vi "RT Proccesing.vi"(8 "error in (no error)":errorcluster, 10 "info":cluster{"File path":T4, "Cfg ":T5} {"Cfg"."Offset_rueda WS 2" format="%.27g"; "Cfg"."Offset_rueda WS 1" format="%.27g"; "Cfg"."Frecuencia de muestreo y módulo CRIO" items=["51.200 kS/s (NI 9234)"=1, "25.600 kS/s (NI 9234)"=2, "17.067 kS/s (NI 9234)"=3, "12.800 kS/s (NI 9234)"=4, "10.240 kS/s (NI 9234)"=5, "8.533 kS/s (NI 9234)"=6, "7.314 kS/s (NI 9234)"=7, "6.400 kS/s (NI 9234)"=8, "5.689 kS/s (NI 9234)"=9, "5.120 kS/s (NI 9234)"=10, "4.654 kS/s (NI 9234)"=11, "4.267 kS/s (NI 9234)"=12, "3.938 kS/s (NI 9234)"=13, "3.657 kS/s (NI 9234)"=14, "3.413 kS/s (NI 9234)"=15, "3.200 kS/s (NI 9234)"=16, "3.012 kS/s (NI 9234)"=17, "2.845 kS/s (NI 9234)"=18, "2.695 kS/s (NI 9234)"=19, "2.560 kS/s (NI 9234)"=20, "2.438 kS/s (NI 9234)"=21, "2.328 kS/s (NI 9234)"=22, "2.226 kS/s (NI 9234)"=23, "2.133 kS/s (NI 9234)"=24, "2.048 kS/s (NI 9234)"=25, "1.969 kS/s (NI 9234)"=26, "1.896 kS/s (NI 9234)"=27, "1.829 kS/s (NI 9234)"=28, "1.765 kS/s (NI 9234)"=29, "1.707 kS/s (NI 9234)"=30, "1.652 kS/s (NI 9234)"=31]}, 11 "Message Queues in":T7) -> (0 "error out":errorcluster)   [LabVIEW 2015]
uses:
  support/Message Queue/All Message Queues.ctl
  support/Message Queue/Message Cluster.ctl
  controls/File paths.ctl
  controls/Cfg_parameters.ctl
  <vilib>/LabVIEW Targets/FPGA/cRIO/shared/nicrio_ModuleControls/nicrio_cRIO-9234_DataRatesRing2.ctl
  controls/Flota.ctl
  controls/Tags.ctl
  controls/Processing data.ctl
  support/Message Queue/Enqueue Message (Single).vi
  <vilib>/Utility/file.llb/Write Delimited Spreadsheet (string).vi
  <vilib>/Utility/error.llb/Error Cluster From Error Code.vi
  <vilib>/ErrorRing/Error Ring.xnode
  support/Message Queue/Message Queue.lvlib
  AURA_Wheel/Json2Labv.lvlib
  AURA_Wheel/AuraWheelAPI/AuraWheel.lvlib
panel:
  out "Response headers":string
  out "data":cluster{"status":string}
  in  "Procesado":T1
  in  "TAGs":T2
  in  "Flota":T3
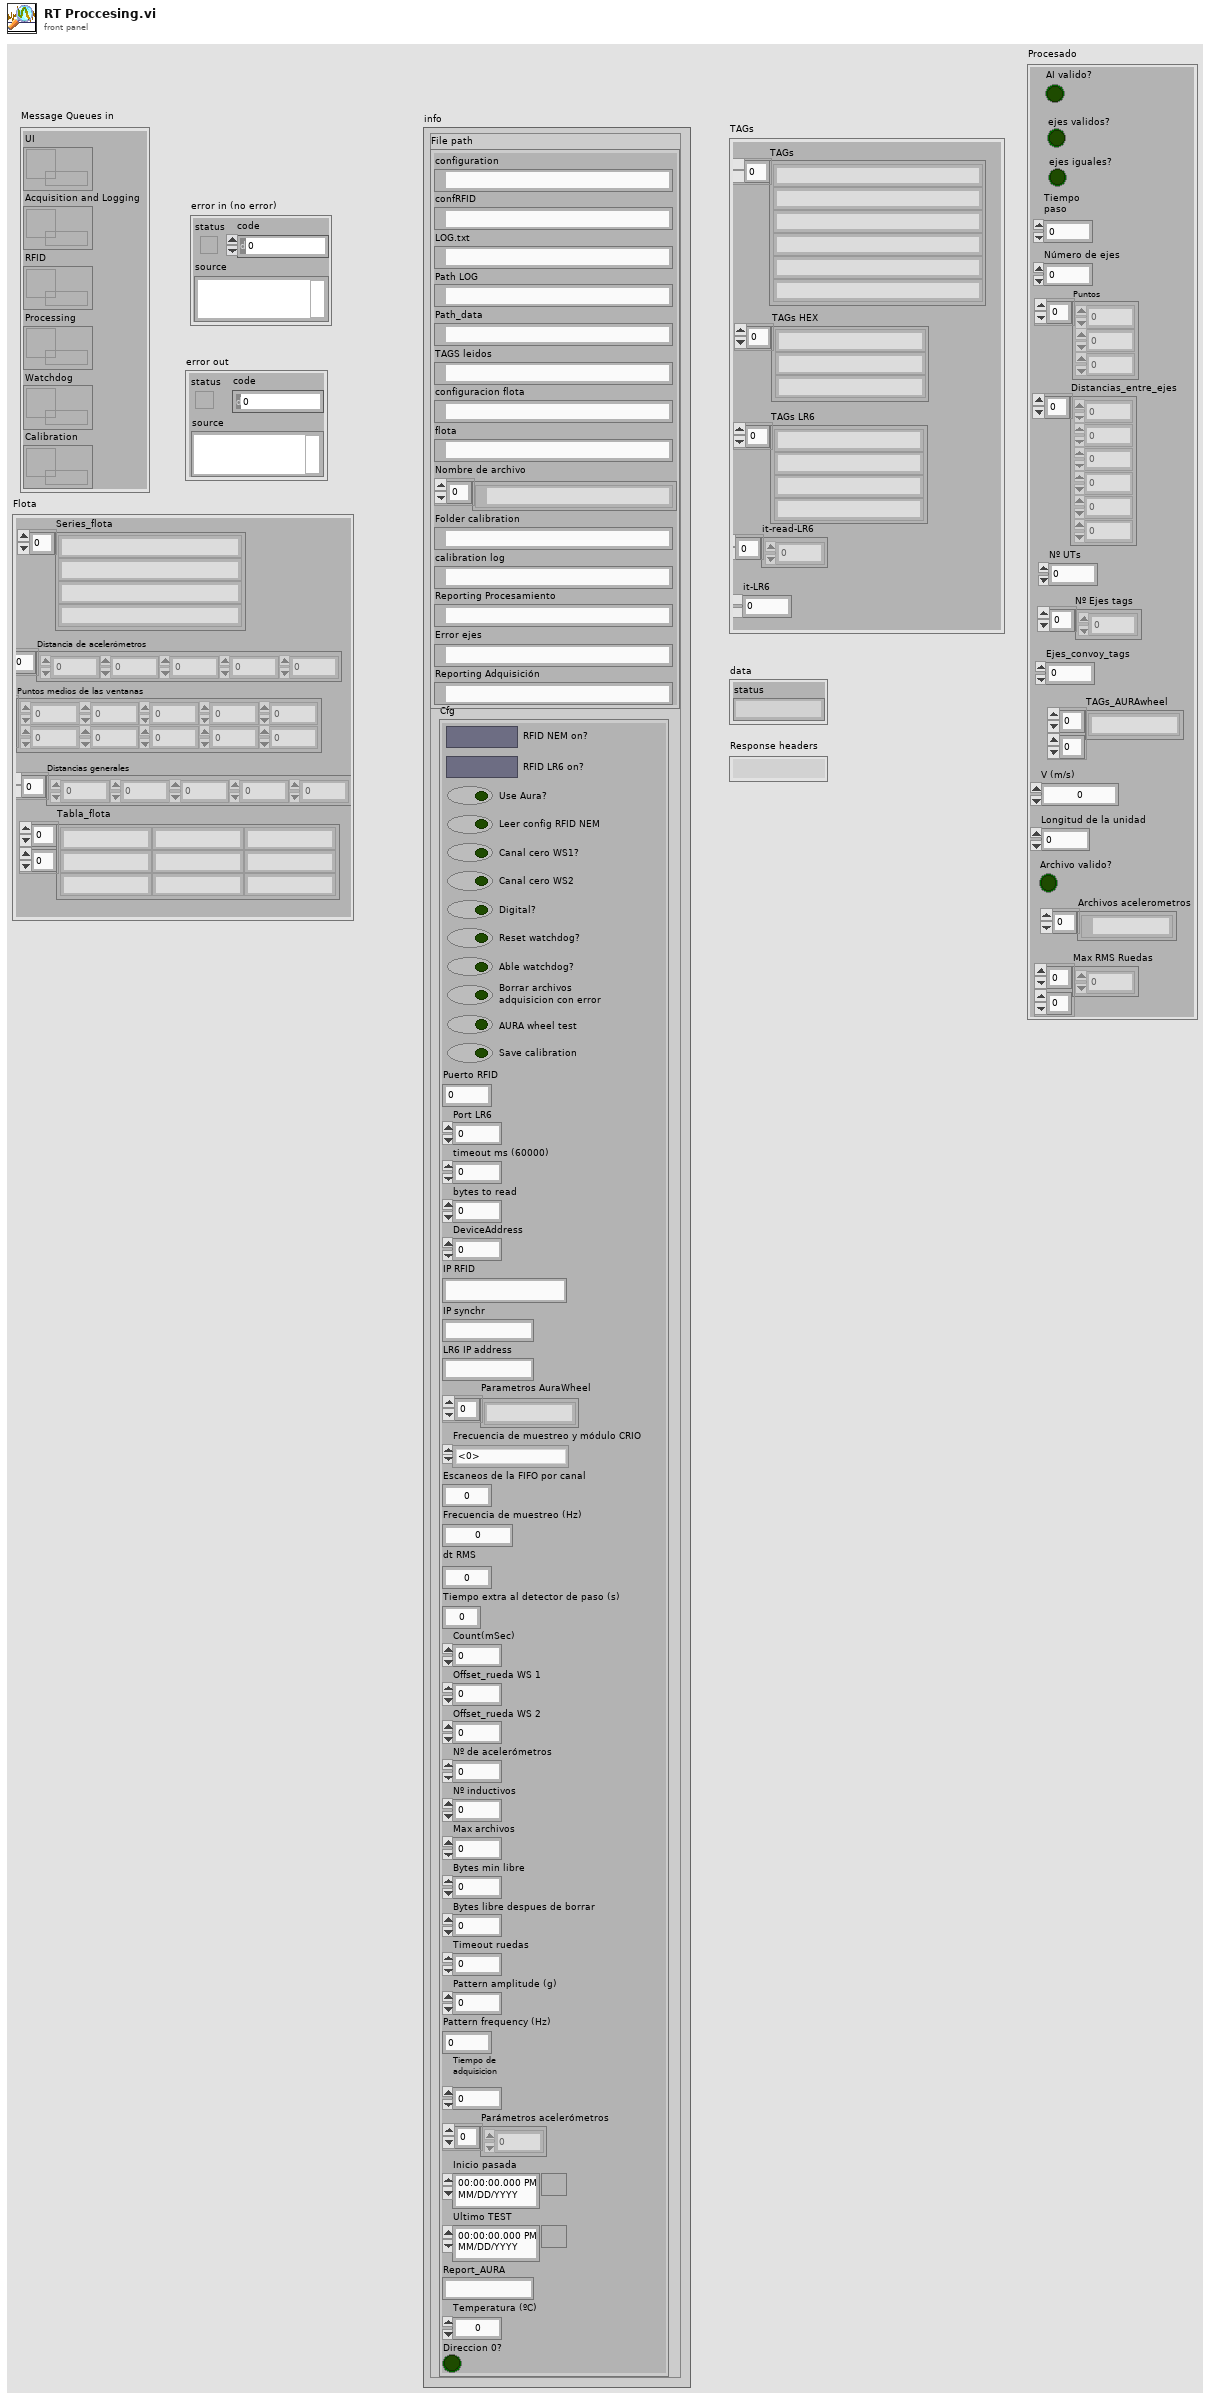
[diagram p1: front panel]
types:
  T1 = typedef "Processing data.ctl" = cluster{"AI valido?":bool, "Tiempo\npaso":dbl, "Puntos":sgl[], "Número de ejes":i32, "ejes validos?":bool, "ejes iguales?":bool, "Distancias_entre_ejes":dbl[], "Nº UTs":i32, "Nº Ejes tags":i32[], "Ejes_convoy_tags":i32, "TAGs_AURAwheel":string[][], "V (m/s)":dbl, "Longitud de la unidad":dbl, "Archivo valido?":bool, "Archivos acelerometros":path[], "Max RMS Ruedas":dbl[][]}
  T2 = typedef "Tags.ctl" = cluster{"TAGs":string[], "TAGs HEX":string[], "TAGs LR6":string[], "it-read-LR6":i32[], "it-LR6":i32}
  T3 = typedef "Flota.ctl" = cluster{"Series_flota":string[], "Distancia de acelerómetros":dbl[], "Puntos medios de las ventanas":dbl[][], "Distancias generales":dbl[], "Tabla_flota":string[][]}
  T4 = typedef "File paths.ctl" = cluster{"configuration":path, "confRFID":path, "LOG.txt":path, "Path LOG":path, "Path_data":path, "TAGS leidos":path, "configuracion flota":path, "flota":path, "Nombre de archivo":path[], "Folder calibration":path, "calibration log":path, "Reporting Procesamiento":path, "Error ejes":path, "Reporting Adquisición":path}
  T5 = typedef "Cfg_parameters.ctl" = cluster{"RFID NEM on?":bool, "RFID LR6 on?":bool, "Use Aura?":bool, "Leer config RFID NEM":bool, "Canal cero WS1?":bool, "Canal cero WS2 ":bool, "Digital?":bool, "Reset watchdog?":bool, "Able watchdog?":bool, "Borrar archivos\nadquisicion con error":bool, "AURA wheel test":bool, "Save calibration":bool, "Puerto RFID":u16, "Port LR6":u16, "timeout ms (60000)":i32, "bytes to read":i32, "DeviceAddress":u8, "IP RFID":string, "IP synchr":string, "LR6 IP address":string, "Parametros AuraWheel":string[], "Frecuencia de muestreo y módulo CRIO":T6, "Escaneos de la FIFO por canal":u32, "Frecuencia de muestreo (Hz)":dbl, "dt RMS":dbl, "Tiempo extra al detector de paso (s)":dbl, "Count(mSec)":u32, "Offset_rueda WS 1":fxp<+/-,24,-4>, "Offset_rueda WS 2":fxp<+/-,24,-4>, "Nº de acelerómetros":i32, "Nº inductivos":i32, "Max archivos":u32, "Bytes min libre":u32, "Bytes libre despues de borrar":u32, "Timeout ruedas":dbl, "Pattern amplitude (g)":dbl, "Pattern frequency (Hz)":dbl, "Tiempo de adquisicion\n":dbl, "Parámetros acelerómetros":dbl[], "Inicio pasada":timestamp, "Ultimo TEST":timestamp, "Report_AURA":string, "Temperatura (ºC)":dbl, "Direccion 0?":bool}
  T6 = typedef "nicrio_cRIO-9234_DataRatesRing2.ctl" = u8
  T7 = typedef "Message Queue.lvlib/All Message Queues.ctl" = cluster{"UI":refnum<queue>, "Acquisition and Logging":refnum<queue>, "RFID":refnum<queue>, "Processing":refnum<queue>, "Watchdog":refnum<queue>, "Calibration":refnum<queue>}
  T8 = enum16{"big-endian, network order", "native, host order", "little-endian"}
  T9 = cluster{"g_ts":dbl, "p_sp":dbl, "p_tp":dbl, "p_tg":cluster{"tg_n":dbl, "tg_t":string}[], "p_ax":cluster{"ax_n":dbl, "ax_sp":dbl, "ax_wh":cluster{"wh_p":dbl, "wh_a1":dbl, "wh_a2":dbl, "wh_a3":dbl, "wh_a4":dbl}[]}[]}
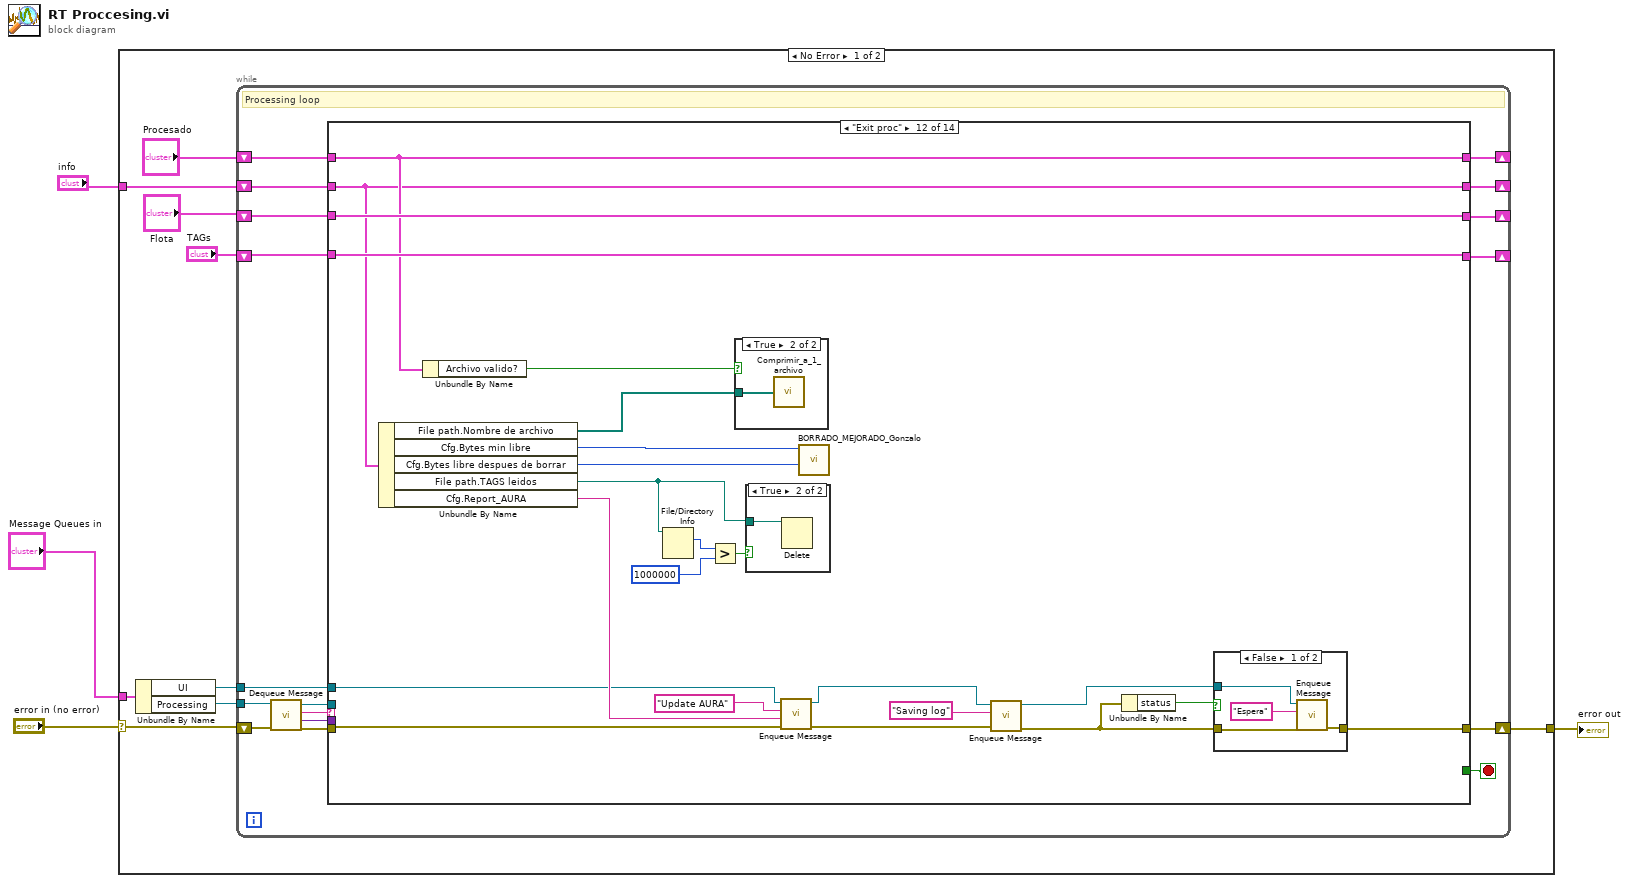
[diagram p0: block diagram]
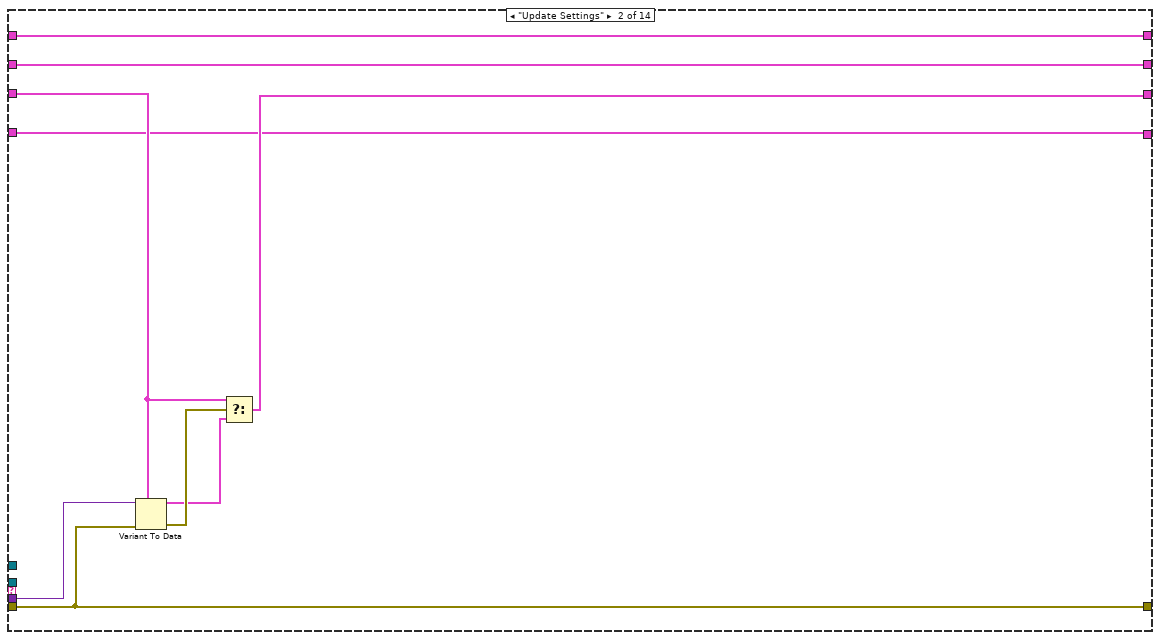
[diagram p3: hidden frame]
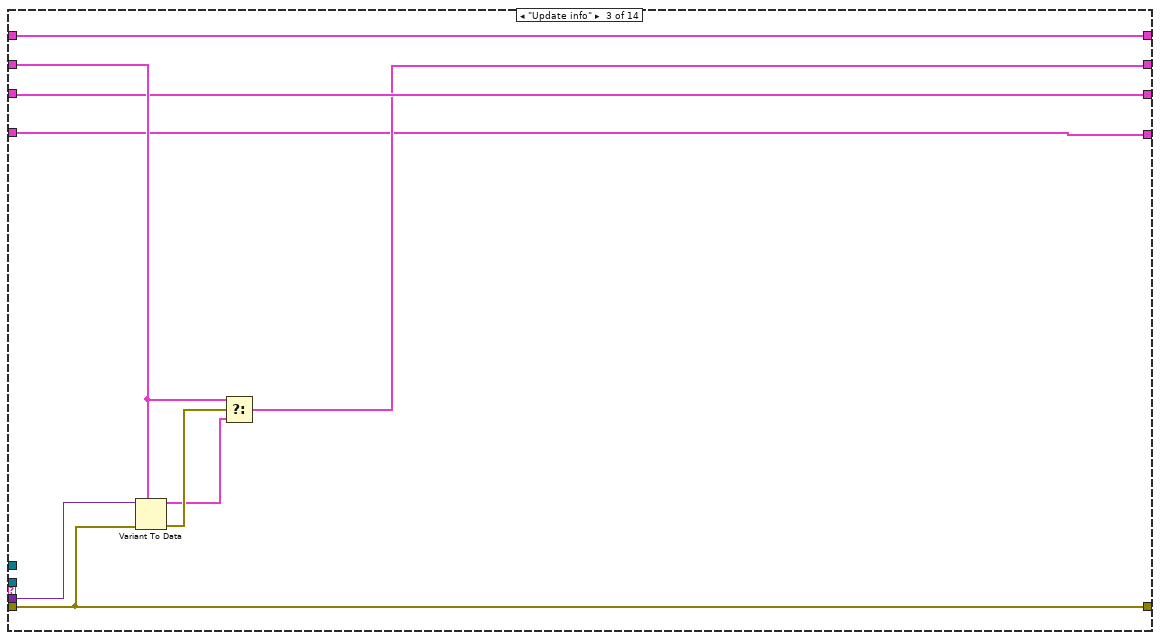
[diagram p4: hidden frame]
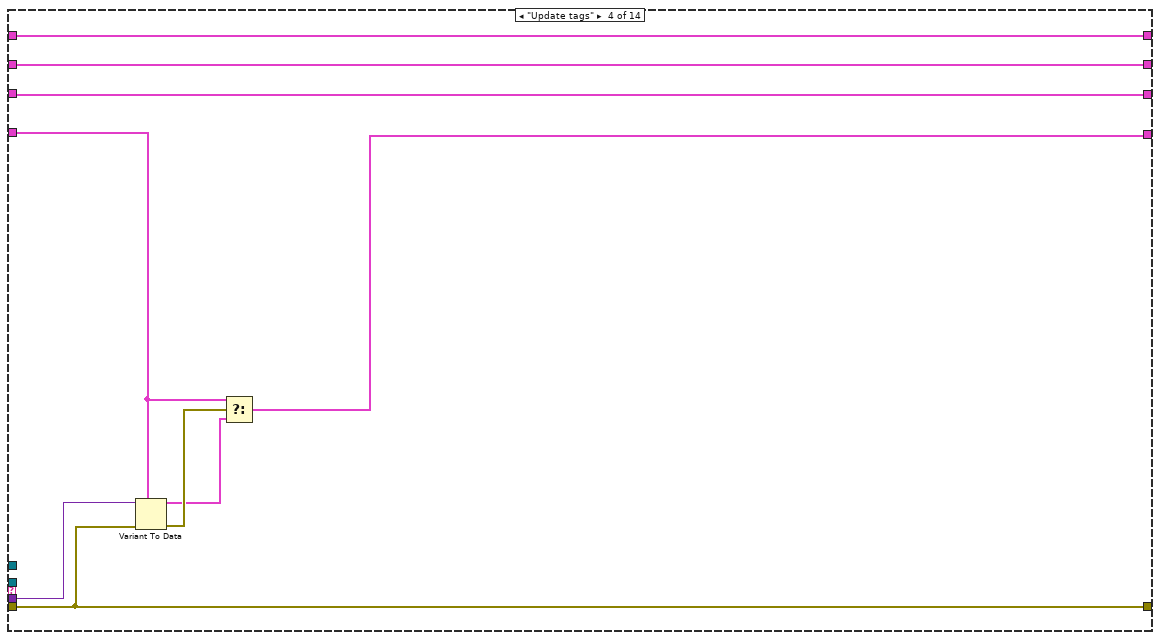
[diagram p5: hidden frame]
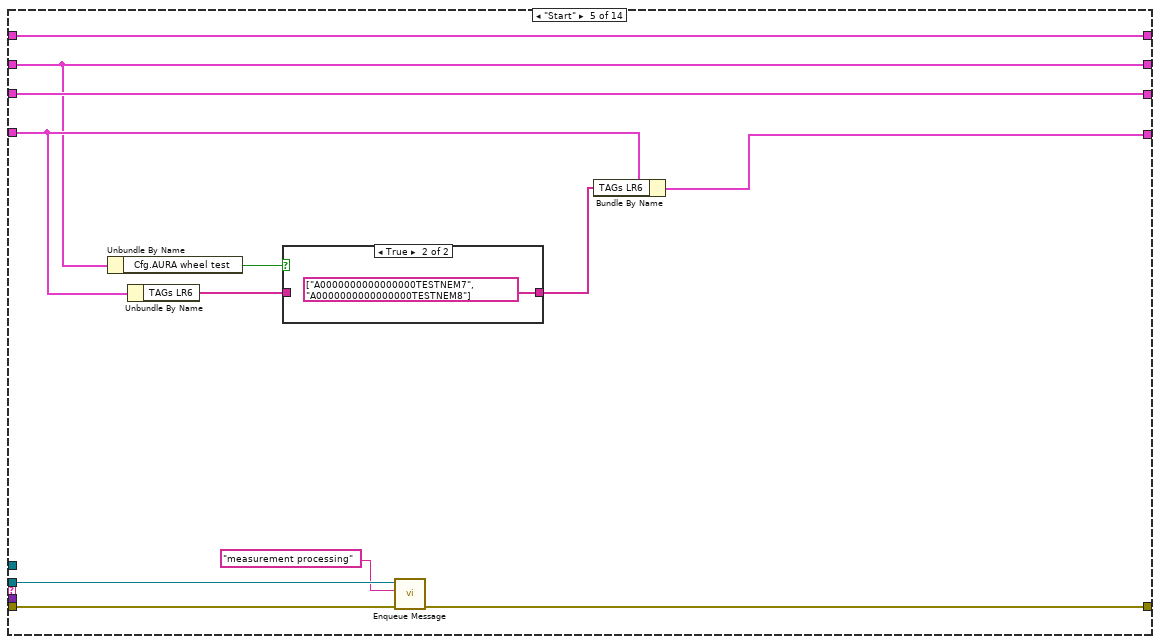
[diagram p6: hidden frame]
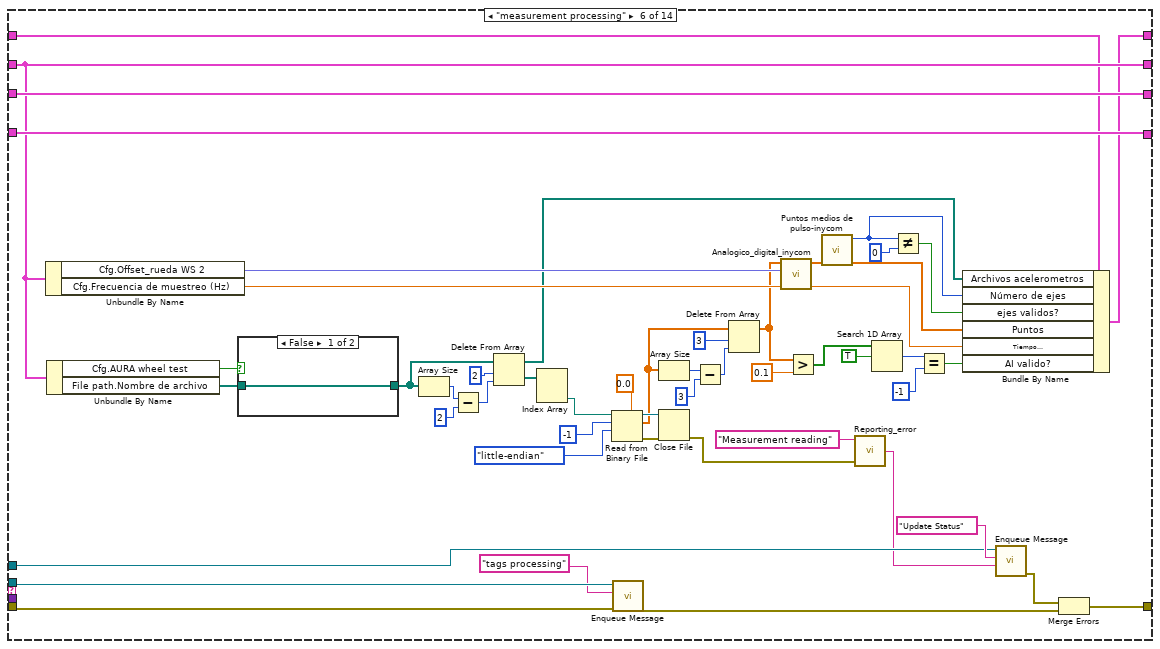
[diagram p8: hidden frame]
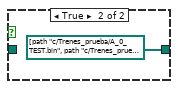
[diagram p9: hidden frame]
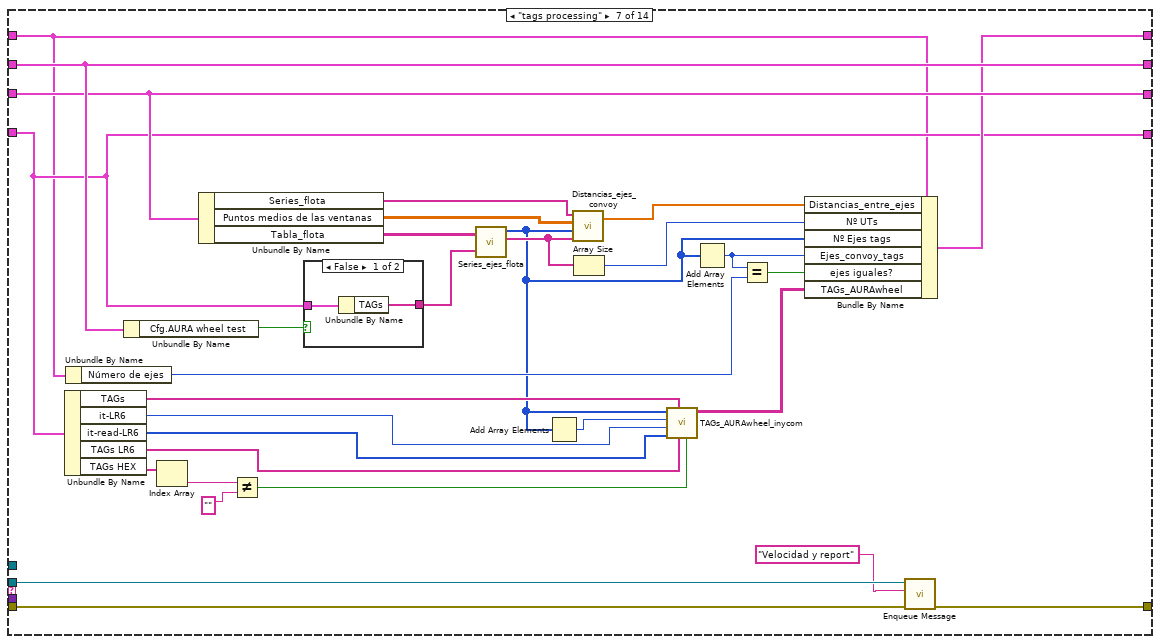
[diagram p10: hidden frame]
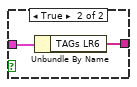
[diagram p11: hidden frame]
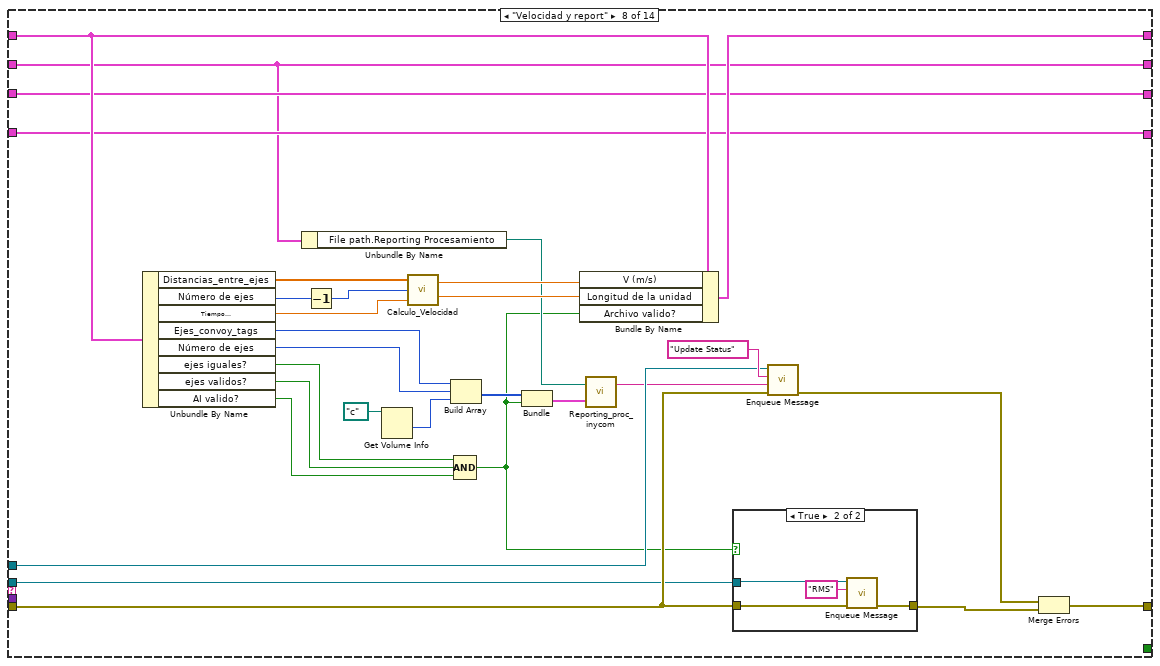
[diagram p12: hidden frame]
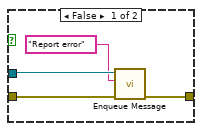
[diagram p13: hidden frame]
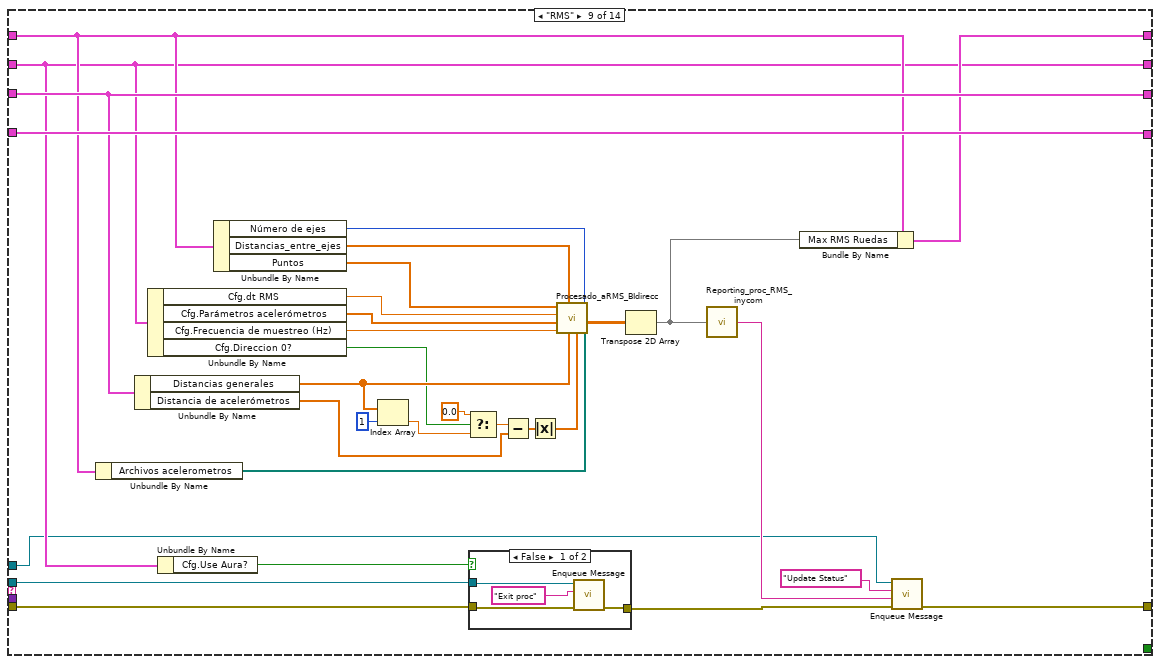
[diagram p14: hidden frame]
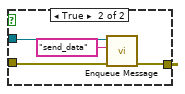
[diagram p15: hidden frame]
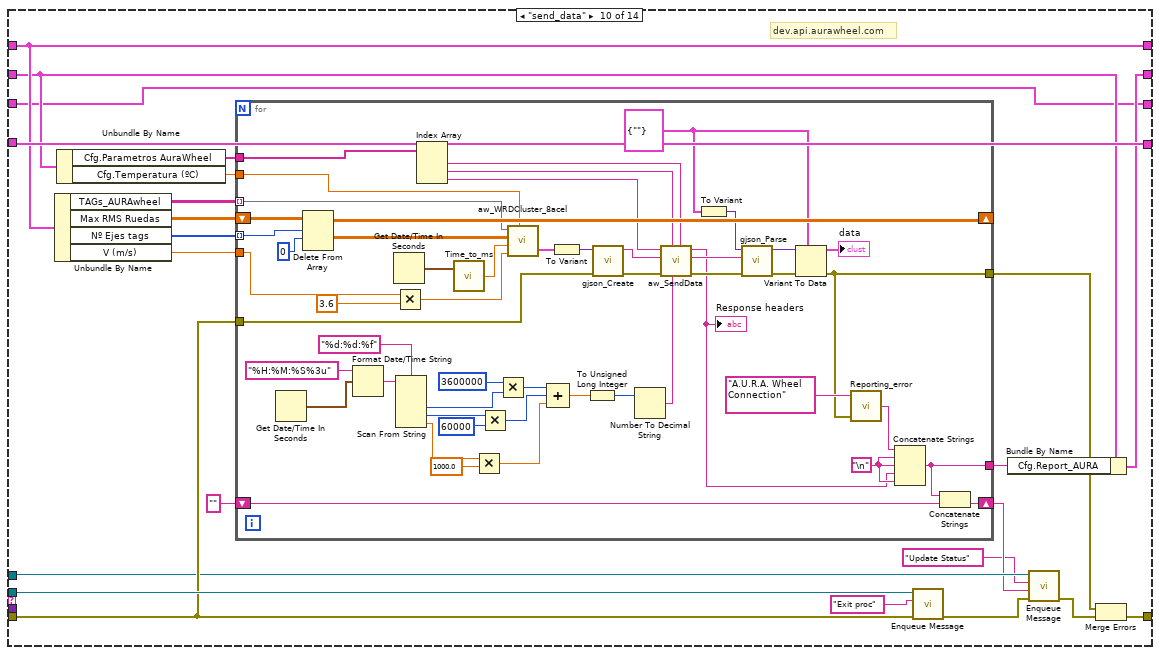
[diagram p16: hidden frame]
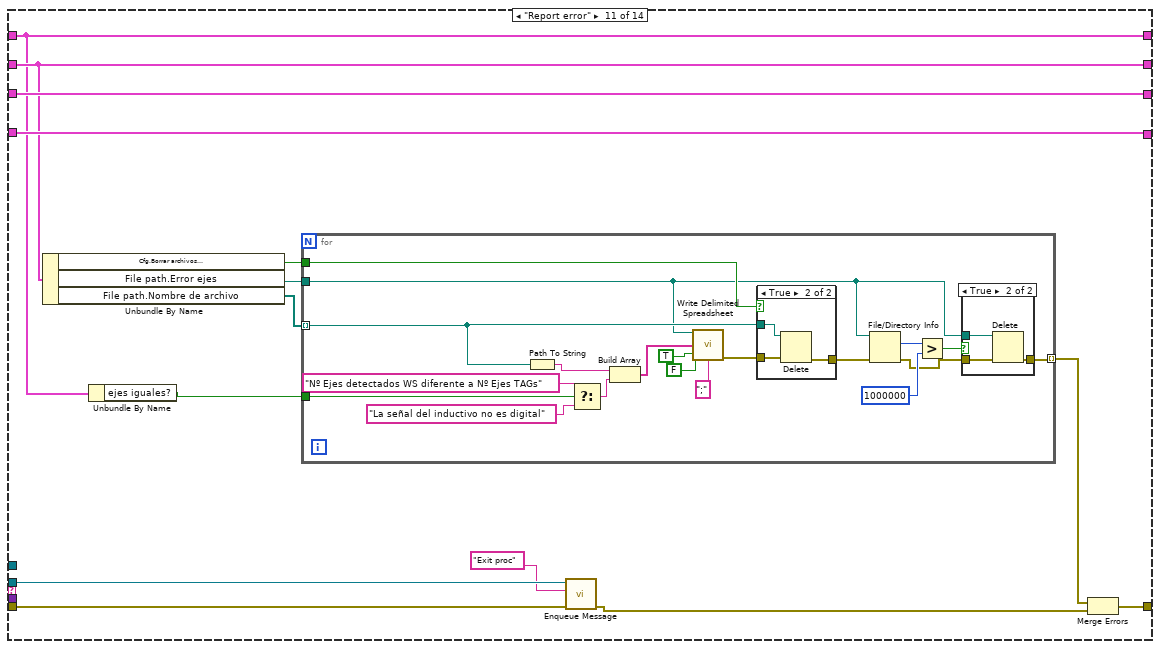
[diagram p17: hidden frame]
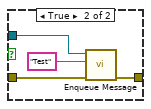
[diagram p20: hidden frame]
diagram:
  n1 = case shown="No Error" "error in (no error)" {
    selector: "error in (no error)" -> [w12 w412]
    tunnel: "Message Queues in" -> [w13 _]
    tunnel: "info" -> [w9 _]
    tunnel: [w8 w412] -> w1
    frame No Error {
      n2 = Unbundle By Name(w13) -> ("UI"=w10:refnum<queue>, "Processing"=w11:refnum<queue>)
      n3 = while {
        tunnel: w11 -> [w29]
        tunnel: w10 -> [w27]
        shift-right: [w23] -> _
        shift-left: w9 -> [w24]
        shift-right: [w19] -> _
        shift-left: "Flota" -> [w20]
        shift-right: [w16] -> _
        shift-left: "TAGs" -> [w17]
        shift-right: [w14] -> _
        shift-left: "Procesado" -> [w15]
        shift-right: [w21] -> w8
        shift-left: w12 -> [w30]
        stop <- w22 stop-if-true
        # "Processing loop"
        n4 = call "Dequeue Message.vi"("error in (no error)"=w30, "Message Queue"=w29) -> ("error out"=w26:errorcluster, "Message Data"=w18:variant, "Message"=w25:string, "dup Message Queue"=w28:refnum<queue>)  [unwired: 6 in]
        n5 = case shown="\"Exit proc\"" w25 {
          selector: w25 -> [_ _ _ _ _ _ _ _ _ _ _ _ _ w402]
          tunnel: w28 -> [_ _ _ _ w65 w97 w133 w169 w209 w262 w318 _ w396 _]
          tunnel: w27 -> [_ _ _ _ _ w99 _ w172 w203 w253 _ w360 _ _]
          tunnel: w26 -> [w35 w38 w50 w59 w74 w96 w132 w170 w211 w255 w320 w365 w397 _]
          tunnel: [w35 w38 w50 w59 w73 w91 w131 w168 w205 w254 w322 w361 w395 w403] -> w21
          tunnel: w24 -> [w34 w44 w49 w57 w66 w94 w159 w179 w212 w248 w328 w377 w398 w404]
          tunnel: [w34 w44 w47 w57 w66 w94 w159 w179 w212 w247 w328 w377 w398 w404] -> w23
          tunnel: [_ _ _ _ _ _ _ _ _ _ _ _ TRUE _] -> w22
          tunnel: w20 -> [w33 w41 w48 w58 w70 w109 w157 w183 w232 w242 w330 w380 w393 w401]
          tunnel: [w33 w39 w48 w58 w70 w109 w157 w183 w232 w242 w330 w380 w393 w401] -> w19
          tunnel: w18 -> [_ w43 w53 w62 _ _ _ _ _ _ _ _ _ _]
          tunnel: [w32 w37 w46 w55 w67 w108 w146 w184 w233 w264 w329 w379 w392 w400] -> w16
          tunnel: w17 -> [w32 w37 w46 w56 w69 w108 w146 w184 w233 w264 w329 w379 w392 w400]
          tunnel: w15 -> [w31 w36 w45 w54 w63 w85 w134 w190 w214 w249 w325 w378 w391 w399]
          tunnel: [w31 w36 w45 w54 w63 w84 w152 w189 w213 w249 w325 w378 w391 w399] -> w14
          frame "Initialize" {
          }
          frame "Update Settings" {
            n6 = Variant To Data(error in=w38, type=w41, Variant=w43) -> (data=w40:T3, error out=w42:errorcluster)
            n7 = Select(t=w41, s=w42, f=w40) -> (s? t:f=w39:T3)
          }
          frame "Update info" {
            n8 = Variant To Data(error in=w50, type=w49, Variant=w53) -> (data=w51:cluster{"File path":T4, "Cfg ":T5}, error out=w52:errorcluster)
            n9 = Select(t=w49, s=w52, f=w51) -> (s? t:f=w47:cluster{"File path":T4, "Cfg ":T5})
          }
          frame "Update tags" {
            n10 = Variant To Data(error in=w59, type=w56, Variant=w62) -> (data=w60:T2, error out=w61:errorcluster)
            n11 = Select(t=w56, s=w61, f=w60) -> (s? t:f=w55:T2)
          }
          frame "Start" {
            n12 = Unbundle By Name(w66) -> ("Cfg.AURA wheel test"=w72:bool)
            n13 = Unbundle By Name(w69) -> ("TAGs LR6"=w71:string[])
            n14 = case shown="True" w72 {
              tunnel: w71 -> [w75 _]
              tunnel: [w75 string[] ["A0000000000000000TESTNEM7", "A0000000000000000TESTNEM8"]] -> w68
              frame False {
              }
              frame True {
              }
            }
            n15 = call-poly "Enqueue Message.vi"("error in (no error)"=w74, "Message"="measurement processing", "Message Queue"=w65) -> ("error out"=w73:errorcluster)  [unwired: 7 in, 1 out]
            n16 = Bundle By Name(cluster=w69, "TAGs LR6"=w68) -> (w67:T2)
          }
          frame "measurement processing" {
            n17 = Unbundle By Name(w94) -> ("Cfg.Offset_rueda WS 2"=w93:fxp<+/-,24,-4>, "Cfg.Frecuencia de muestreo (Hz)"=w92:dbl)
            n18 = Unbundle By Name(w94) -> ("Cfg.AURA wheel test"=w127:bool, "File path.Nombre de archivo"=w126:path[])
            n19 = case shown="False" w127 {
              tunnel: w126 -> [w128 _]
              tunnel: [w128 path[] [path "c:/Trenes_prueba/A_0_TEST.bin", path "c:/Trenes_prueba/A_1_TEST.bin", path "c:/Trenes_prueba/A_2_TEST.bin", path "c:/Trenes_prueba/A_3_TEST.bin", path "c:/Trenes_prueba/A_4_TEST.bin", path "c:/Trenes_prueba/A_5_TEST.bin", path "c:/Trenes_prueba/A_6_TEST.bin", path "c:/Trenes_prueba/A_7_TEST.bin", path "c:/Trenes_prueba/I_0_TEST.bin", path "c:/Trenes_prueba/I_1_TEST.bin"]] -> w110
              frame False {
              }
              frame True {
              }
            }
            n20 = Array Size(array=w110) -> (size(s)=w123:i32)
            n21 = Subtract(x=w123, y=2 ("length")) -> (x-y=w125:i32)
            n22 = Delete From Array(array=w110, length=2, index=w125) -> (deleted portion=w112:path[], array with subset deleted=w78:path[])
            n23 = Index Array(array=w112) -> (element #2=w111:path)  [unwired: 2 in, 1 out]
            n24 = Read from Binary File(5:sgl 0.0, 9:T8."little-endian" ("byte order (0:big-endian, network order)"), 10:-1 ("count (1)"), 11:w111) -> (0:w121:errorcluster, 2:w95:sgl[], 3:w122:refnum<file>)  [unwired: 1 in, 2 out]
            n25 = call-poly "Enqueue Message.vi"("error in (no error)"=w96, "Message"="tags processing", "Message Queue"=w97) -> ("error out"=w89:errorcluster)  [unwired: 7 in, 1 out]
            n26 = Array Size(array=w95) -> (size(s)=w117:i32)
            n27 = Close File(refnum=w122, error in=w121) -> (error out=w101:errorcluster)  [unwired: 1 out]
            n28 = Subtract(x=w117, y=3 ("length")) -> (x-y=w115:i32)
            n29 = Delete From Array(array=w95, length=3, index=w115) -> (array with subset deleted=w77:sgl[])  [unwired: 1 out]
            n30 = call "Analogico_digital_inycom.vi"("Frecuencia muestreo"=w92, "Offset WS"=w93, "Array"=w77) -> ("Tiempo\npaso"=w82:dbl, "array out"=w87:sgl[])  [unwired: 7 in]
            n31 = Greater?(x=w77, y=0.1) -> (0:w104:bool[])
            n32 = call "Puntos medios de pulso-inycom.vi"("DI Inductivo"=w87) -> ("Puntos"=w81:sgl[], "Número de ejes"=w79:i32)  [unwired: 9 in]
            n33 = call "Reporting_error.vi"("error out 2"=w101, "Concept"="Measurement reading") -> ("Reporting"=w98:string)  [unwired: 1 in]
            n34 = Search 1D Array(1D array=w104, element=TRUE) -> (index of element=w106:i32)  [unwired: 1 in]
            n35 = Not Equal?(x=w79, y=0) -> (x != y?=w80:bool)
            n36 = Equal?(x=w106, y=-1) -> (x = y?=w83:bool)
            n37 = Bundle By Name(cluster=w85, "Archivos acelerometros"=w78, "Número de ejes"=w79, "ejes validos?"=w80, "Puntos"=w81, "Tiempo\npaso"=w82, "AI valido?"=w83) -> (w84:T1)
            n38 = call-poly "Enqueue Message.vi"("Message Data"=w98, "Message"="Update Status", "Message Queue"=w99) -> ("error out"=w90:errorcluster)  [unwired: 7 in, 1 out]
            n39 = Merge Errors(w90, w89) -> (w91:errorcluster)
          }
          frame "tags processing" {
            n40 = Unbundle By Name(w146) -> ("TAGs"=w144:string[], "it-LR6"=w141:i32, "it-read-LR6"=w140:i32[], "TAGs LR6"=w136:string[], "TAGs HEX"=w138:string[])
            n41 = Unbundle By Name(w134) -> ("Número de ejes"=w148:i32)
            n42 = Unbundle By Name(w159) -> ("Cfg.AURA wheel test"=w160:bool)
            n43 = Index Array(array=w138) -> (element=w137:string)  [unwired: 1 in]
            n44 = Unbundle By Name(w157) -> ("Series_flota"=w154:string[], "Puntos medios de las ventanas"=w155:dbl[][], "Tabla_flota"=w156:string[][])
            n45 = Not Equal?(x=w137, y="" ("delimiter (\\t)")) -> (x != y?=w139:bool)
            n46 = case shown="False" w160 {
              tunnel: w146 -> [w162 w164]
              tunnel: [w161 w163] -> w158
              frame False {
                n47 = Unbundle By Name(w162) -> ("TAGs"=w161:string[])
              }
              frame True {
                n48 = Unbundle By Name(w164) -> ("TAGs LR6"=w163:string[])
              }
            }
            n49 = call "Series_ejes_flota.vi"("Tabla_flota"=w156, "Tags"=w158) -> ("Nº Ejes"=w143:i32[], "Series del convoy"=w151:string[])  [unwired: 2 in, 1 out]
            n50 = Add Array Elements(numeric array=w143) -> (sum=w142:i32)
            n51 = call "Distancias_ejes_convoy.vi"("Series_flota1"=w151, "Ejes_UT"=w143, "Puntos medios de las ventanas"=w155, "Series_flota"=w154) -> ("Distancias_entre_ejes_convoy"=w153:dbl[])  [unwired: 1 in]
            n52 = Array Size(array=w151) -> (size(s)=w150:i32)
            n53 = call "TAGs_AURAwheel_inycom.vi"("Plataformas?"=w139, "TAGs LR6"=w136, "TAGs"=w144, "it-read-LR6"=w140, "it-LR6"=w141, "Ejes_convoy"=w142, "Nº Ejes"=w143) -> ("TAGS_AURA"=w135:string[][])  [unwired: 4 in]
            n54 = Add Array Elements(numeric array=w143) -> (sum=w149:i32)
            n55 = Equal?(x=w149, y=w148) -> (x = y?=w147:bool)
            n56 = Bundle By Name(cluster=w134, "Distancias_entre_ejes"=w153, "Nº UTs"=w150, "Nº Ejes tags"=w143, "Ejes_convoy_tags"=w149, "ejes iguales?"=w147, "TAGs_AURAwheel"=w135) -> (w152:T1)
            n57 = call-poly "Enqueue Message.vi"("error in (no error)"=w132, "Message"="Velocidad y report", "Message Queue"=w133) -> ("error out"=w131:errorcluster)  [unwired: 7 in, 1 out]
          }
          frame "Velocidad y report" {
            n58 = Unbundle By Name(w190) -> ("Distancias_entre_ejes"=w194:dbl[], "Número de ejes"=w193:i32, "Tiempo\npaso"=w191:dbl, "Ejes_convoy_tags"=w182:i32, "Número de ejes"=w181:i32, "ejes iguales?"=w176:bool, "ejes validos?"=w175:bool, "AI valido?"=w174:bool)
            n59 = Unbundle By Name(w179) -> ("File path.Reporting Procesamiento"=w178:path)
            n60 = Decrement(x=w193) -> (x-1=w192:i32)
            n61 = Get Volume Info(11:path "c:/" ("path")) -> (1:w185:i64)  [unwired: 1 in, 5 out]
            n62 = call "Calculo_Velocidad.vi"("Tiempo de paso (s)"=w191, "Ejes"=w192, "Puntos iniciales de las ventanas"=w194) -> ("V (m/s)"=w187:dbl, "Longitud de la unidad"=w188:dbl)
            n63 = Build Array(w182, w181, w185) -> (w177:i64[])
            n64 = Compound Arithmetic op=AND(w176, w175, w174) -> (w165:bool)
            n65 = Bundle(w177, w165) -> (w180:cluster{i64[], bool})  [unwired: 1 in]
            n66 = Bundle By Name(cluster=w190, "V (m/s)"=w188, "Longitud de la unidad"=w187, "Archivo valido?"=w165) -> (w189:T1)
            n67 = call "Reporting_proc_inycom.vi"("cluster"=w180, "address repoting"=w178) -> ("Reporting"=w171:string)  [unwired: 1 in]
            n68 = case shown="True" w165 {
              tunnel: w170 -> [w197 w202]
              tunnel: w169 -> [w196 w200]
              tunnel: [w198 w201] -> w167
              frame False {
                n69 = call-poly "Enqueue Message.vi"("error in (no error)"=w197, "Message"="Report error", "Message Queue"=w196) -> ("error out"=w198:errorcluster)  [unwired: 7 in, 1 out]
              }
              frame True {
                n70 = call-poly "Enqueue Message.vi"("error in (no error)"=w202, "Message"="RMS", "Message Queue"=w200) -> ("error out"=w201:errorcluster)  [unwired: 7 in, 1 out]
              }
            }
            n71 = call-poly "Enqueue Message.vi"("error in (no error)"=w170, "Message Data"=w171, "Message"="Update Status", "Message Queue"=w172) -> ("error out"=w166:errorcluster)  [unwired: 6 in, 1 out]
            n72 = Merge Errors(w166, w167) -> (w168:errorcluster)
          }
          frame "RMS" {
            n73 = Unbundle By Name(w214) -> ("Archivos acelerometros"=w216:path[])
            n74 = Unbundle By Name(w232) -> ("Distancias generales"=w225:dbl[], "Distancia de acelerómetros"=w218:dbl[])
            n75 = Unbundle By Name(w212) -> ("Cfg.dt RMS"=w228:dbl, "Cfg.Parámetros acelerómetros"=w227:dbl[], "Cfg.Frecuencia de muestreo (Hz)"=w226:dbl, "Cfg.Direccion 0?"=w222:bool)
            n76 = Unbundle By Name(w212) -> ("Cfg.Use Aura?"=w210:bool)
            n77 = Unbundle By Name(w214) -> ("Número de ejes"=w231:i32, "Distancias_entre_ejes"=w230:dbl[], "Puntos"=w229:sgl[])
            n78 = Index Array(array=w225, index=1) -> (element=w221:dbl)
            n79 = Select(t=0.0, s=w222, f=w221) -> (s? t:f=w219:dbl)
            n80 = case shown="False" w210 {
              tunnel: w211 -> [w237 w241]
              tunnel: w209 -> [w235 w239]
              tunnel: [w236 w240] -> w206
              frame False {
                n81 = call-poly "Enqueue Message.vi"("error in (no error)"=w237, "Message"="Exit proc", "Message Queue"=w235) -> ("error out"=w236:errorcluster)  [unwired: 7 in, 1 out]
              }
              frame True {
                n82 = call-poly "Enqueue Message.vi"("error in (no error)"=w241, "Message"="send_data", "Message Queue"=w239) -> ("error out"=w240:errorcluster)  [unwired: 7 in, 1 out]
              }
            }
            n83 = Subtract(x=w219, y=w218) -> (x-y=w220:dbl[])
            n84 = Absolute Value(x=w220) -> (abs(x)=w217:dbl[])
            n85 = call "Procesado_aRMS_BIdirecc.vi"("Paths_canales_aRMS"=w216, "Ejes Procesados"=w231, "Distancias\nacelerometros"=w217, "Distancias generales (m)"=w225, "Distancias centrales de las ruedas\n               configuración (m)"=w230, "Frecuencia de muestreo"=w226, "Parámetros acelerómetros"=w227, "dt RMS 2"=w228, "Puntos"=w229) -> ("Max RMS Ruedas"=w215:dbl[][])  [unwired: 2 in]
            n86 = Transpose 2D Array(2D array=w215) -> (transposed array=w208:dbl[][])
            n87 = call "Reporting_proc_RMS_inycom.vi"("Max RMS Ruedas"=w208) -> ("String"=w204:string)
            n88 = Bundle By Name(cluster=w214, "Max RMS Ruedas"=w208) -> (w213:T1)
            n89 = call-poly "Enqueue Message.vi"("error in (no error)"=w206, "Message Data"=w204, "Message"="Update Status", "Message Queue"=w203) -> ("error out"=w205:errorcluster)  [unwired: 6 in, 1 out]
          }
          frame "send_data" {
            # "dev.api.aurawheel.com"
            n90 = Unbundle By Name(w249) -> ("TAGs_AURAwheel"=w261:string[][], "Max RMS Ruedas"=w260:dbl[][], "Nº Ejes tags"=w259:i32[], "V (m/s)"=w258:dbl)
            n91 = Unbundle By Name(w248) -> ("Cfg.Parametros AuraWheel"=w256:string[], "Cfg.Temperatura (ºC)"=w257:dbl)
            n92 = for {
              tunnel: w256 -> [w316]
              tunnel: w261 -> [w310] mode=indexing
              shift-right: [w312] -> _
              shift-left: w260 -> [w314]
              tunnel: w259 -> [w313] mode=indexing
              tunnel: w258 -> [w306]
              tunnel: w257 -> [w304]
              tunnel: w255 -> [w297]
              tunnel: [w268] -> w250
              tunnel: [w266] -> w246
              shift-right: [w267] -> w244
              shift-left: "" -> [w265]
              w272 = "\n"
              w274 = cluster{"status":string} {"status"=""}
              n93 = Get Date/Time In Seconds() -> (seconds since 1Jan1904=w293:timestamp)
              n94 = Delete From Array(array=w314, length=w313, index (row)=0) -> (deleted portion=w309:dbl[][], array with subset deleted=w312:dbl[][])  [unwired: 1 in]
              n95 = Format Date/Time String(time format string (%c)="%H:%M:%S%3u", seconds (now)=w293) -> (date/time string=w291:string)  [unwired: 1 in]
              n96 = Get Date/Time In Seconds() -> (seconds since 1Jan1904=w311:timestamp)
              n97 = Multiply(x=w306, y=3.6) -> (x*y=w305:dbl)
              n98 = Scan From String(format string="%d:%d:%f", input string=w291) -> (output 1=w288:i32, output 2=w287:i32, output 3=w280:dbl)  [unwired: 5 in, 3 out]
              n99 = Index Array(array=w316) -> (element #1=w294:string, element #2=w295:string, element #3=w296:string)  [unwired: 3 in]
              n100 = call "Time_to_ms.vi"("seconds since 1Jan1904"=w311) -> ("Numeric"=w308:dbl)  [unwired: 1 in]
              n101 = Multiply(x=w280, y=1000.0) -> (x*y=w281:dbl)
              n102 = Multiply(x=w287, y=60000) -> (x*y=w284:i32)
              n103 = Multiply(x=3600000, y=w288) -> (x*y=w285:i32)
              n104 = call "aw_WRDCluster_8acel.vi"("Array TAGs"=w310, "Max RMS Ruedas"=w309, "TimeStamp"=w308, "p_sp"=w305, "p_tp"=w304) -> ("JSON cluster"=w298:T9)  [unwired: 1 in]
              n105 = Compound Arithmetic op=ADD(w285, w284, w281) -> (w283:dbl)
              n106 = To Variant(anything=w298) -> (Variant=w303:variant)
              n107 = To Unsigned Long Integer(number=w283) -> (unsigned 32bit integer=w282:u32)
              n108 = call "gjson_Create.vi"("error in"=w297, "JSON Object in"=w303) -> ("error out"=w301:errorcluster, "JSON String Out"=w302:string)  [unwired: 8 in]
              n109 = Number To Decimal String(number=w282) -> (decimal integer string=w278:string)  [unwired: 1 in]
              n110 = call "aw_SendData.vi"("pwd"=w294, "x-nem-datetime"=w278, "User"=w295, "error in"=w301, "JSON Object"=w302, "URL"=w296) -> ("error out"=w299:errorcluster, "Response JSON"=w300:string, "Response headers"=w269:string)  [unwired: 3 in]
              "Response headers" <- w269
              n111 = To Variant(anything=w274) -> (Variant=w277:variant)
              n112 = call "gjson_Parse.vi"("error in"=w299, "JSON String In"=w300, "JSON Cluster"=w277) -> ("error out"=w276:errorcluster, "JSON Cluster Out"=w275:variant)  [unwired: 7 in]
              n113 = Variant To Data(error in=w276, type=w274, Variant=w275) -> (data=→"data":cluster{"status":string}, error out=w268:errorcluster)
              n114 = call "Reporting_error.vi"("error out 2"=w268, "Concept"="A.U.R.A. Wheel Connection") -> ("Reporting"=w270:string)  [unwired: 1 in]
              n115 = Concatenate Strings(w270, w272, w272, w269, w272) -> (w266:string)
              n116 = Concatenate Strings(w266, w265) -> (w267:string)
            }
            n117 = call-poly "Enqueue Message.vi"("error in (no error)"=w255, "Message"="Exit proc", "Message Queue"=w262) -> ("error out"=w251:errorcluster)  [unwired: 7 in, 1 out]
            n118 = Bundle By Name(cluster=w248, "Cfg.Report_AURA"=w246) -> (w247:cluster{"File path":T4, "Cfg ":T5})
            n119 = call-poly "Enqueue Message.vi"("error in (no error)"=w251, "Message Data"=w244, "Message"="Update Status", "Message Queue"=w253) -> ("error out"=w252:errorcluster)  [unwired: 6 in, 1 out]
            n120 = Merge Errors(w250, w252) -> (w254:errorcluster)
          }
          frame "Report error" {
            n121 = Unbundle By Name(w328) -> ("Cfg.Borrar archivos\nadquisicion con error"=w323:bool, "File path.Error ejes"=w327:path, "File path.Nombre de archivo"=w326:path[])
            n122 = Unbundle By Name(w325) -> ("ejes iguales?"=w324:bool)
            n123 = for {
              tunnel: w327 -> [w331]
              tunnel: w326 -> [w338] mode=indexing
              tunnel: w324 -> [w341]
              tunnel: w323 -> [w340]
              tunnel: [w334] -> w321 mode=indexing
              n124 = Path To String(path=w338) -> (string=w346:string)
              n125 = Select(t="Nº Ejes detectados WS diferente a Nº Ejes TAGs" ("delimiter (\\t)"), s=w341, f="La señal del inductivo no es digital" ("delimiter (\\t)")) -> (s? t:f=w343:string)
              n126 = Build Array(w346, w343) -> (w342:string[])
              n127 = call-poly <vilib>:"Write Delimited Spreadsheet.vi"("file path (dialog if empty)"=w331, "1D data"=w342, "append to file? (F)"=FALSE ("transpose? (no:F)"), "transpose? (F)"=TRUE ("append to file? (new file:F)"), "delimiter (\\t)"=";" ("delimiter (\\t)")) -> ("error out"=w339:errorcluster)  [unwired: 9 in, 1 out]
              n128 = case shown="True" w340 {
                tunnel: w339 -> [w354 w357]
                tunnel: [w354 w356] -> w332
                tunnel: w338 -> [_ w355]
                frame False {
                }
                frame True {
                  n129 = Delete(path (use dialog)=w355, error in=w357) -> (error out=w356:errorcluster)  [unwired: 5 out]
                }
              }
              n130 = File/Directory Info(path=w331, error in=w332) -> (size=w337:i64, error out=w333:errorcluster)  [unwired: 5 out]
              n131 = Greater?(x=w337, y=i64 1000000) -> (0:w335:bool)
              n132 = case shown="True" w335 {
                tunnel: w331 -> [_ w353]
                tunnel: w333 -> [w350 w352]
                tunnel: [w350 w351] -> w334
                frame False {
                }
                frame True {
                  n133 = Delete(path (use dialog)=w353, error in=w352) -> (error out=w351:errorcluster)  [unwired: 3 in, 2 out]
                }
              }
            }
            n134 = call-poly "Enqueue Message.vi"("error in (no error)"=w320, "Message"="Exit proc", "Message Queue"=w318) -> ("error out"=w319:errorcluster)  [unwired: 7 in, 1 out]
            n135 = Merge Errors(w321, w319) -> (w322:errorcluster)
          }
          frame "Exit proc" {
            n136 = Unbundle By Name(w377) -> ("File path.Nombre de archivo"=w375:path[], "Cfg.Bytes min libre"=w374:u32, "Cfg.Bytes libre despues de borrar"=w373:u32, "File path.TAGS leidos"=w369:path, "Cfg.Report_AURA"=w364:string)
            n137 = Unbundle By Name(w378) -> ("Archivo valido?"=w376:bool)
            n138 = File/Directory Info(path=w369) -> (size=w372:i64)  [unwired: 1 in, 6 out]
            n139 = Greater?(x=w372, y=i64 1000000) -> (0:w370:bool)
            n140 = case shown="True" w376 {
              tunnel: w375 -> [_ w390]
              frame False {
              }
              frame True {
                n141 = call "Comprimir_a_1_archivo.vi"("Acel_paths"=w390) -> ()  [unwired: 1 out]
              }
            }
            n142 = case shown="True" w370 {
              tunnel: w369 -> [_ w389]
              frame False {
              }
              frame True {
                n143 = Delete(path (use dialog)=w389) -> ()  [unwired: 4 in, 3 out]
              }
            }
            n144 = call-poly "Enqueue Message.vi"("error in (no error)"=w365, "Message Data"=w364, "Message"="Update AURA", "Message Queue"=w360) -> ("error out"=w366:errorcluster, "dup Message Queue"=w359:refnum<queue>)  [unwired: 6 in]
            n145 = call "BORRADO_MEJORADO_Gonzalo.vi"("Bytes LIBRE OK"=w373, "Bytes Minimo de Memoria libre"=w374) -> ()  [unwired: 10 in]
            n146 = call-poly "Enqueue Message.vi"("error in (no error)"=w366, "Message"="Saving log", "Message Queue"=w359) -> ("error out"=w362:errorcluster, "dup Message Queue"=w358:refnum<queue>)  [unwired: 7 in]
            n147 = Unbundle By Name(w362) -> ("status"=w363:bool)
            n148 = case shown="False" w363 {
              tunnel: w358 -> [w381 w388]
              tunnel: w362 -> [w383 w387]
              tunnel: [w382 w386] -> w361
              frame False {
                n149 = call-poly "Enqueue Message.vi"("error in (no error)"=w383, "Message"="Espera", "Message Queue"=w381) -> ("error out"=w382:errorcluster)  [unwired: 7 in, 1 out]
              }
              frame True {
                n150 = call-poly "Enqueue Message.vi"("error in (no error)"=w387, "Message"="Test", "Message Queue"=w388) -> ("error out"=w386:errorcluster)  [unwired: 7 in, 1 out]
              }
            }
          }
          frame "Exit" {
            n151 = Release Queue(queue=w396, error in (no error)=w397) -> (error out=w395:errorcluster)  [unwired: 1 in, 2 out]
          }
          frame Default {
            n152 = xnode "Error Ring"("parameter 0"=w402) -> ("error out"=w403:errorcluster)
          }
        }
      }
    }
    frame Error {
    }
  }
  "error out" <- w1
